vi "Build Frame Name from Category and State.vi"(7 "Wrap in Quotes? (TRUE)":bool, 10 "State Name":string, 11 "Category":string) -> (3 "Frame Name":string)   [LabVIEW 2020, in "JKI State Machine API.lvlib" / "JKI SM.lvclass"]
uses:
  JKI SM.lvclass
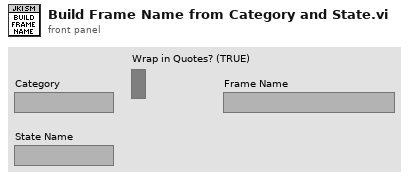
[diagram p1: front panel]
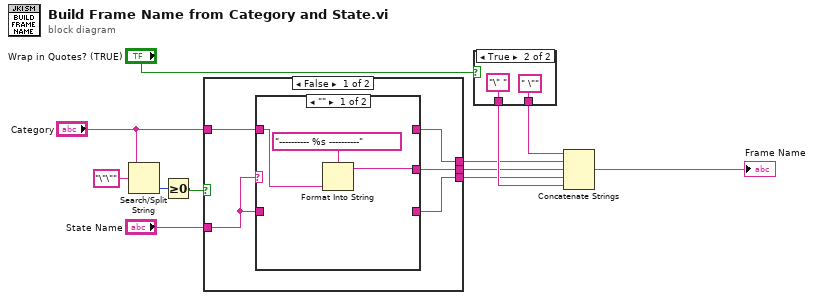
[diagram p0: block diagram]
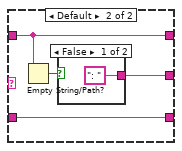
[diagram p2: hidden frame]
diagram:
  n1 = Search/Split String(string="Category", search string/char (-)="\"\"") -> (offset of match=w3:i32)  [unwired: 1 in, 2 out]
  n2 = Greater Or Equal To 0?(x=w3) -> (x >= 0?=w1:bool)
  n3 = case shown="False" w1 {
    tunnel: [w17 w26] -> w9
    tunnel: [w16 _] -> w7
    tunnel: [w15 _] -> w6
    tunnel: "State Name" -> [w14 _]
    tunnel: "Category" -> [w13 w26]
    frame False {
      n4 = case shown="\"\"" w14 {
        tunnel: [w18 w24] -> w17
        tunnel: w13 -> [w19 w22]
        tunnel: [_ w22] -> w16
        tunnel: [_ w21] -> w15
        tunnel: w14 -> [_ w21]
        frame "" {
          n5 = Format Into String(format string="---------- %s ----------", w19) -> (resulting string=w18:string)  [unwired: 2 in, 1 out]
        }
        frame Default {
          n6 = Empty String/Path?(string/path=w22) -> (empty?=w23:bool)
          n7 = case shown="False" w23 {
            tunnel: [": " ("string") _] -> w24
            frame False {
            }
            frame True {
            }
          }
        }
      }
    }
    frame True {
      # "Is the Idle \"\" frame?"
    }
  }
  n8 = case shown="True" "Wrap in Quotes? (TRUE)" {
    tunnel: [_ "\" " ("string")] -> w12
    tunnel: [_ " \"" ("string")] -> w11
    frame False {
    }
    frame True {
    }
  }
  n9 = Concatenate Strings(w11, w7, w9, w6, w12) -> (→"Frame Name":string)
